vi "Read.vi"(8 "error in (no error)":errorcluster, 11 "VISA Refnum in":refnum<visa-resource-name>) -> (0 "error out":errorcluster, 2 "Read value":string, 3 "VISA Refnum out":refnum<visa-resource-name>)   [LabVIEW 2023, in "Serial_communication.lvlib"]
uses:
  Serial_communication.lvlib
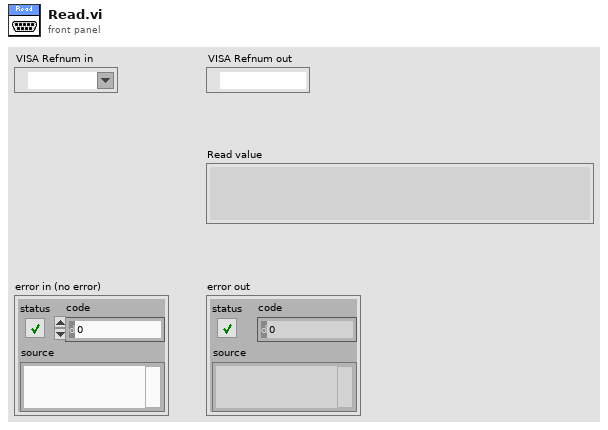
[diagram p1: front panel]
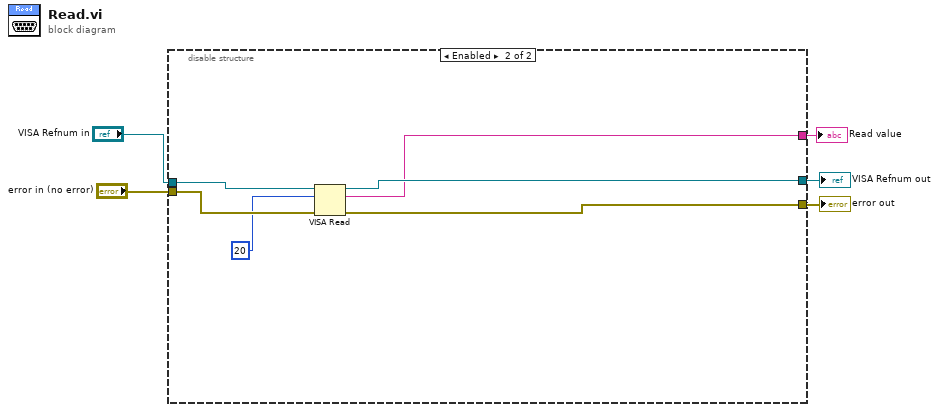
[diagram p0: block diagram]
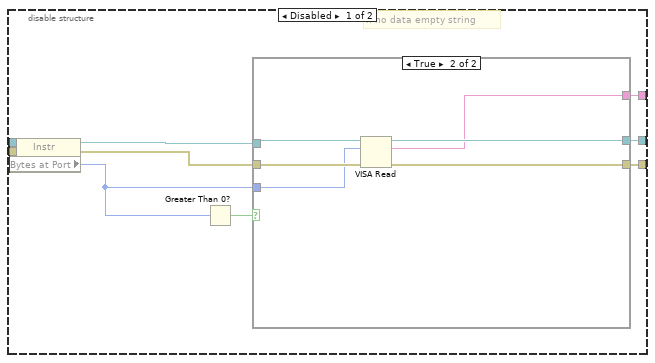
[diagram p2: hidden frame]
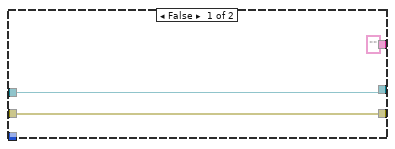
[diagram p3: hidden frame]
diagram:
  n1 = disable-structure shown="Enabled" {
    disable-tunnel: [w14 w25] -> w5
    disable-tunnel: [w13 w28] -> w4
    disable-tunnel: "error in (no error)" -> [w11 w26]
    disable-tunnel: "VISA Refnum in" -> [w10 w29]
    disable-tunnel: [w6 w27] -> w1
    frame Disabled {
      # "if no data empty string"
      n2 = property class="Instr"(reference=w10, error in=w11) -> (reference out=w8:refnum<visa-resource-name>, error out=w7:errorcluster, "Bytes at Port"=w12:u32)
      n3 = Greater Than 0?(x=w12) -> (x > 0?=w9:bool)
      n4 = case shown="True" w9 {
        tunnel: w7 -> [w16 w23]
        tunnel: w8 -> [w17 w22]
        tunnel: [w17 w21] -> w13
        tunnel: [w16 w20] -> w14
        tunnel: w12 -> [_ w19]
        tunnel: ["" ("read buffer") w18] -> w6
        frame False {
        }
        frame True {
          n5 = VISA Read(VISA resource name=w22, byte count=w19, error in (no error)=w23) -> (VISA resource name out=w21:refnum<visa-resource-name>, read buffer=w18:string, error out=w20:errorcluster)  [unwired: 1 out]
        }
      }
    }
    frame Enabled {
      n6 = VISA Read(VISA resource name=w29, byte count=u32 20, error in (no error)=w26) -> (VISA resource name out=w28:refnum<visa-resource-name>, read buffer=w27:string, error out=w25:errorcluster)  [unwired: 1 out]
    }
  }
  "error out" <- w5
  "VISA Refnum out" <- w4
  "Read value" <- w1
